vi "hse-application_GetApplicationPaths.vi"(8 "error in":errorcluster) -> (0 "error out":errorcluster, 1 "Data Directory":path, 2 "Config Directory":path, 3 "Application Directory":path, 4 "Application Base Path":path, 5 "Config/Unit Directory":path, 7 "Tmp Directory":path)   [LabVIEW 2014, in "hse-application.lvclass"]
doc: "Returns the various paths of the hse-lib based application's folder structure:\n- Application Directory (the folder on disk the startup.vi or the .exe is stored in)\n- Config Directory (the folder containing all the configuration files)\n- Data Directory (the folder designed to hold data generated by the application)\n- Config/Unit Directory (the folder holding the configuration for this unit - see config.ini file)\n- Tmp Directory (the system-specific temporary location)\n\nThe <b>Application Base Path</b> points to the root of the call chain. In the development environment, this path is identical to the Application Directory. In a built .exe, this path points to the .exe itself.\n\n\n____\nHAMPEL SOFTWARE ENGINEERING v0.12.0 (2018-09-13 18:21)"
uses:
  hse-application.lvclass
  hse-application.lvclass/hse-application.ctl
  <vilib>/Utility/sysdir.llb/System Directory Type.ctl
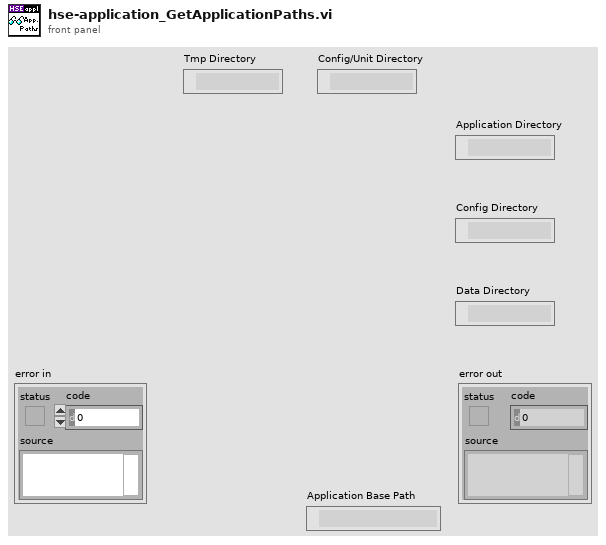
[diagram p1: front panel]
types:
  T1 = typedef "System Directory Type.ctl" = i32
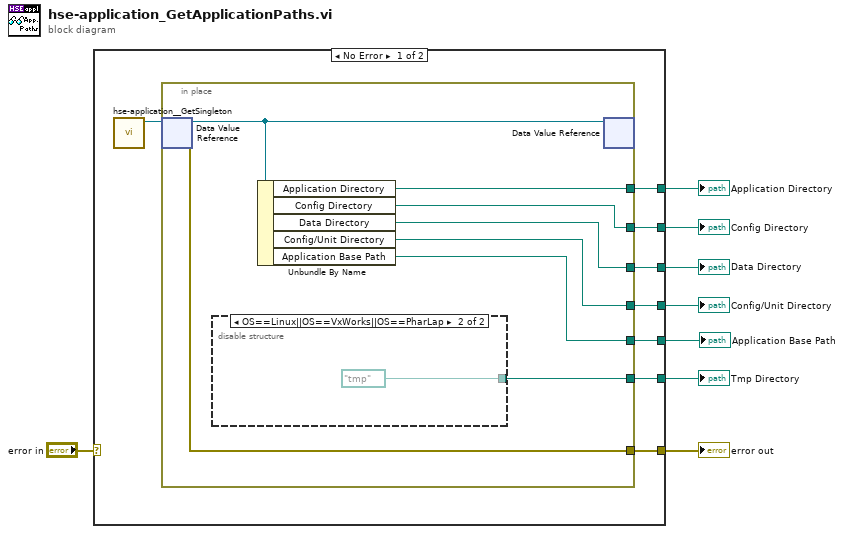
[diagram p0: block diagram]
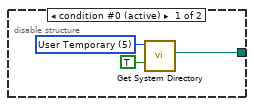
[diagram p2: hidden frame]
diagram:
  n1 = case shown="No Error" "error in" {
    selector: "error in" -> [_ w29]
    tunnel: [w13 w29] -> w7
    tunnel: [w16 _] -> w6
    tunnel: [w15 _] -> w5
    tunnel: [w12 _] -> w4
    tunnel: [w11 _] -> w3
    tunnel: [w10 _] -> w2
    tunnel: [w9 _] -> w1
    frame No Error {
      n2 = call "hse-application__GetSingleton.vi"() -> ("ApplicationClass DVR"=w14:refnum<data-value>)  [unwired: 10 in, 1 out]
      n3 = in-place {
        in-place-border: [w24] -> w16
        in-place-border: [w23] -> w15
        in-place-border: [w21] -> w13
        in-place-border: [w20] -> w12
        in-place-border: [w19] -> w11
        in-place-border: [w18] -> w10
        in-place-border: [w17] -> w9
        n4 = in-place-dvr #1(w14) -> (w22:refnum<class "hse-application.lvclass">, w21:errorcluster)
        n5 = disable-structure shown="OS==Linux||OS==VxWorks||OS==PharLap" {
          disable-tunnel: [w25 path "/tmp" ("system directory")] -> w18
          frame condition #0 (active) {
            w27 = T1 5 items=["User Home"=0, "User Desktop"=1, "User Documents"=2, "User Application Data"=3, "User Preferences"=4, "User Temporary"=5, "Public Documents"=6, "Public Application Data"=7, "Public Preferences"=8, "Public Cache"=13, "System Core Libraries"=9, "System Installed Libraries"=10, "Application Files"=11, "Boot Volume Root"=12] ("system directory type")
            n6 = call <vilib>:"Get System Directory.vi"("create directory if not found? (F)"=TRUE, "system directory type"=w27) -> ("system directory"=w25:path)  [unwired: 9 in]
          }
          frame condition #1 {
          }
        }
        n7 = Unbundle By Name(w22) -> ("Application Directory"=w24:path, "Config Directory"=w23:path, "Data Directory"=w19:path, "Config/Unit Directory"=w20:path, "Application Base Path"=w17:path)
        n8 = in-place-dvr #1(w22) -> ()  [unwired: 2 out]
      }
    }
    frame Error {
    }
  }
  "error out" <- w7
  "Application Directory" <- w6
  "Config Directory" <- w5
  "Config/Unit Directory" <- w4
  "Tmp Directory" <- w2
  "Data Directory" <- w3
  "Application Base Path" <- w1
